vi "Add Object Parameter - Known Type.vi"(5 "JSON Compatible Type":T1=enum."Unknown", 6 "Add Parameter as JSON Tree?":bool, 7 "JSON Type":T2=enum."Unknown", 8 "error in (no error)":errorcluster, 9 "Name":string, 10 "Value":variant, 11 "JSON Tree in (JSON Object)":variant) -> (0 "error out":errorcluster, 3 "JSON Tree out (JSON Object)":variant)   [LabVIEW 2010, in "i3-json.lvlib"]
doc: "Use this template to build a VI to use as a subVI."
uses:
  i3-json.lvlib
  JSON Types/JSON Type.ctl
  JSON Types/JSON Compatible Type.ctl
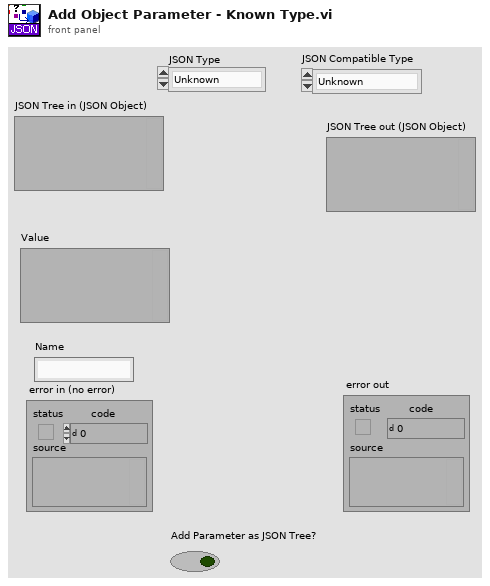
[diagram p1: front panel]
types:
  T1 = typedef "i3-json.lvlib/JSON Compatible Type.ctl" = enum16{"1D Double Array", "1D String Array", "1D Boolean Array", "Unknown"}
  T2 = typedef "i3-json.lvlib/JSON Type.ctl" = enum8{"JSON Compatible", "JSON Array", "JSON Object", "JSON Null", "Double", "String", "Boolean", "Unknown"}
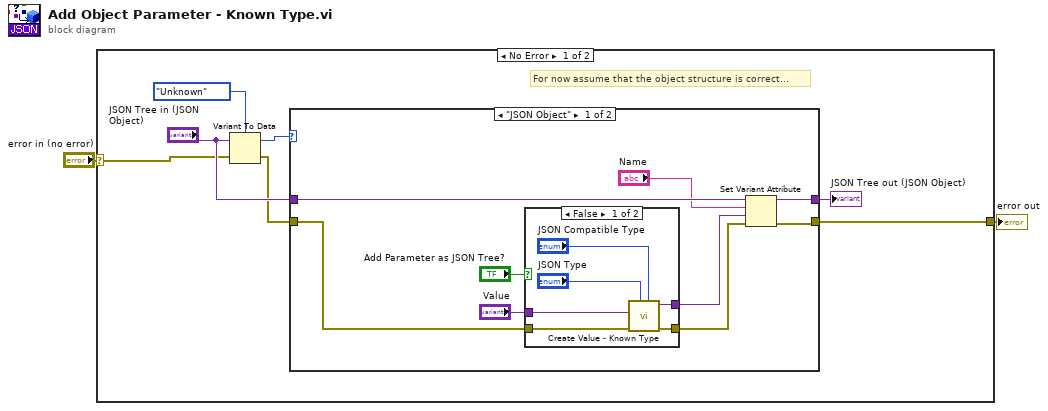
[diagram p0: block diagram]
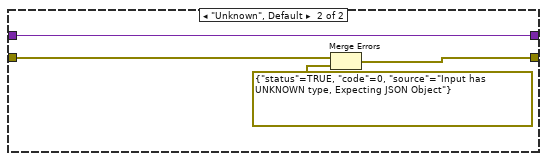
[diagram p3: hidden frame]
diagram:
  n1 = case shown="No Error" "error in (no error)" {
    selector: "error in (no error)" -> [w6 w31]
    tunnel: [w4 w31] -> w1
    frame No Error {
      # "For now assume that the object structure is correct..."
      n2 = Variant To Data(error in=w6, Variant="JSON Tree in (JSON Object)", type=JSON_Type."Unknown" ("JSON Type")) -> (error out=w3:errorcluster, data=w8:T2)
      n3 = case shown="\"JSON Object\"" w8 {
        tunnel: "JSON Tree in (JSON Object)" -> [w13 w30]
        tunnel: w3 -> [w14 w29]
        tunnel: [w16 w30] -> w5
        tunnel: [w15 w28] -> w4
        frame "JSON Object" {
          n4 = case shown="False" "Add Parameter as JSON Tree?" {
            tunnel: [w22 w25] -> w18
            tunnel: [w21 w26] -> w17
            tunnel: w14 -> [w20 w25]
            tunnel: "Value" -> [w19 w26]
            frame False {
              n5 = call "Create Value - Known Type.vi"("JSON Compatible Type"="JSON Compatible Type", "JSON Type"="JSON Type", "error in (no error)"=w20, "Value"=w19) -> ("error out"=w22:errorcluster, "JSON Tree"=w21:variant)  [unwired: 6 in]
            }
            frame True {
              # "ASSUMES VALID JSON\nTREE - maybe Run-Time\ntype check?"
            }
          }
          n6 = Set Variant Attribute(Variant=w13, name="Name", value=w17, error in=w18) -> (Variant out=w16:variant, error out=w15:errorcluster)  [unwired: 1 out]
        }
        frame "Unknown", Default {
          n7 = Merge Errors(w29, errorcluster {"status"=TRUE, "code"=0, "source"="Input has UNKNOWN type, Expecting JSON Object"} ("error in")) -> (w28:errorcluster)
        }
      }
      "JSON Tree out (JSON Object)" <- w5
    }
    frame Error {
    }
  }
  "error out" <- w1
